vi "DriveSimulationInit.vi"() -> (1 "Module Positions":T6[](array[typedef]) {"Angle"."SIN" format="%13.4f"; "Angle"."COS" format="%13.4f"; "Angle"."VALUE" format="%13.4f"}, 2 "TravelMotorDmd":dbl, 3 "SWERVE_DRIVE_KINEMATICS":T1 {"SavedModuleStates"."Angle"."SIN" format="%13.4f"; "SavedModuleStates"."Angle"."COS" format="%13.4f"; "SavedModuleStates"."Angle"."VALUE" format="%13.4f"; "PrevCoR"."Y" format="%14.3f"; "PrevCoR"."X" format="%14.3f"; "Modules"."Y" format="%14.3f"; "Modules"."X" format="%14.3f"})   [LabVIEW 2023]
uses:
  <vilib>/Rock Robotics/WPI/ThirdParty/JAS_Junk/TrajLib/Trajectory_Library.lvlib
  DriveGlobal.vi
  <vilib>/Rock Robotics/WPI/ThirdParty/JAS_Junk/TrajLib/TypeDef/ROTATION2D.ctl
  <vilib>/Rock Robotics/WPI/ThirdParty/JAS_Junk/TrajLib/TypeDef/SWERVE_DRIVE_MODULE_POSITION.ctl
  <vilib>/Analysis/Matrix/Datatypes/RealMatrix.ctl
  <vilib>/Analysis/Matrix/NI_Matrix.lvlib
  <vilib>/Rock Robotics/WPI/ThirdParty/JAS_Junk/TrajLib/TypeDef/TRANSLATION2D.ctl
  <vilib>/Rock Robotics/WPI/ThirdParty/JAS_Junk/TrajLib/TypeDef/SWERVE_DRIVE_MODULE_STATE.ctl
  <vilib>/Rock Robotics/WPI/ThirdParty/JAS_Junk/TrajLib/TypeDef/SWERVE_DRIVE_KINEMATICS.ctl
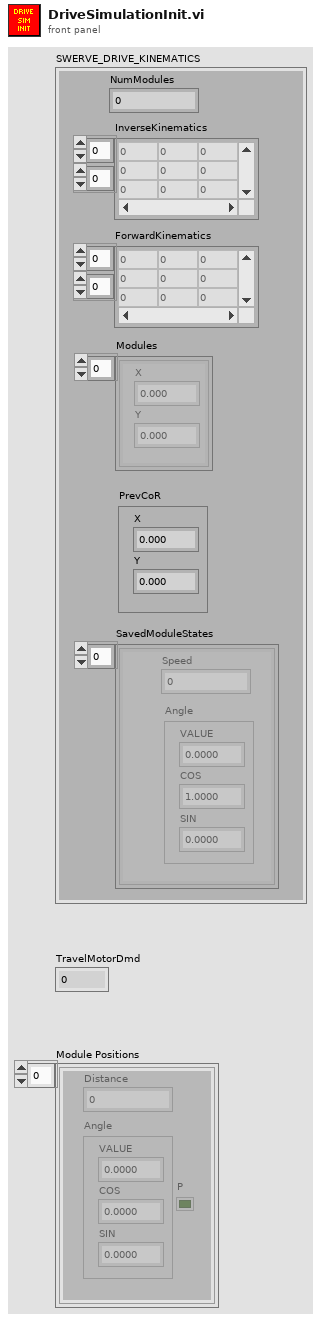
[diagram p1: front panel]
types:
  T1 = typedef "Trajectory_Library.lvlib/SWERVE_DRIVE_KINEMATICS.ctl" = cluster{"NumModules":i32, "InverseKinematics":T2, "ForwardKinematics":T2, "Modules":T3[], "PrevCoR":T3, "SavedModuleStates":T4[]}
  T2 = typedef "NI_Matrix.lvlib/RealMatrix.ctl" = dbl[][]
  T3 = typedef "Trajectory_Library.lvlib/TRANSLATION2D.ctl" = cluster{"X":dbl, "Y":dbl}
  T4 = typedef "Trajectory_Library.lvlib/SWERVE_DRIVE_MODULE_STATE.ctl" = cluster{"Speed":dbl, "Angle":T5}
  T5 = typedef "Trajectory_Library.lvlib/ROTATION2D.ctl" = cluster{"VALUE":dbl, "COS":dbl, "SIN":dbl}
  T6 = typedef "Trajectory_Library.lvlib/SWERVE_DRIVE_MODULE_POSITION.ctl" = cluster{"Distance":dbl, "Angle":T5, "P":bool}
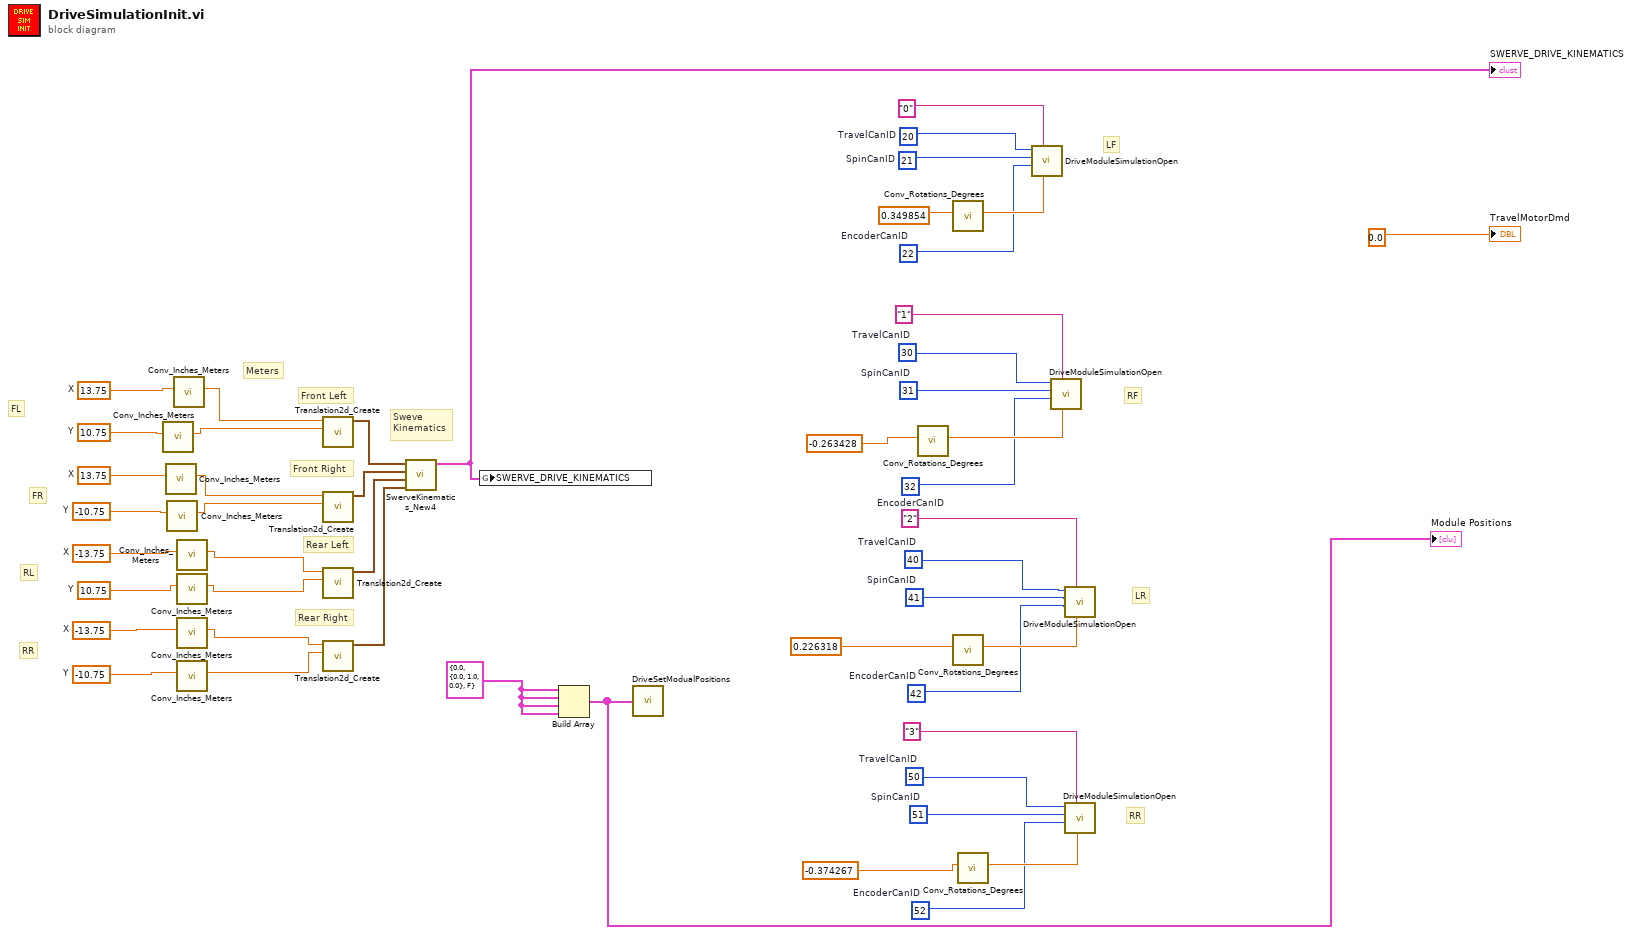
[diagram p0: block diagram]
diagram:
  w36 = u8 50  # TravelCanID
  w37 = u8 51  # SpinCanID
  w38 = u8 52  # EncoderCanID
  w33 = u8 40  # TravelCanID
  w34 = u8 41  # SpinCanID
  w35 = u8 42  # EncoderCanID
  w30 = u8 30  # TravelCanID
  w31 = u8 31  # SpinCanID
  w32 = u8 32  # EncoderCanID
  w29 = u8 20  # TravelCanID
  w28 = u8 21  # SpinCanID
  w27 = u8 22  # EncoderCanID
  w21 = T6 {"Distance"=0.0, "Angle"={"VALUE"=0.0, "COS"=1.0, "SIN"=0.0}, "P"=FALSE} ("SWERVE_DRIVE_MODULE_POSITION")
  w19 = -13.75  # X
  w20 = -10.75  # Y
  w17 = -13.75  # X
  w18 = 10.75  # Y
  w15 = 13.75  # X
  w16 = -10.75  # Y
  w13 = 13.75  # X
  w14 = 10.75  # Y
  # "RR"
  # "LR"
  # "RF"
  # "LF"
  # "RR"
  # "RL"
  # "FR"
  # "FL"
  # "Meters"
  # "Sweve\nKinematics"
  # "Rear Right"
  # "Rear Left"
  # "Front Right"
  # "Front Left"
  n1 = call <vilib>:"Conv_Inches_Meters.vi"("INCH"=w14) -> ("Meters"=w11:dbl)  [unwired: 10 in]
  n2 = call <vilib>:"Conv_Inches_Meters.vi"("INCH"=w15) -> ("Meters"=w10:dbl)  [unwired: 10 in]
  n3 = call <vilib>:"Conv_Inches_Meters.vi"("INCH"=w16) -> ("Meters"=w9:dbl)  [unwired: 10 in]
  n4 = call <vilib>:"Conv_Inches_Meters.vi"("INCH"=w13) -> ("Meters"=w12:dbl)  [unwired: 10 in]
  n5 = call <vilib>:"Conv_Inches_Meters.vi"("INCH"=w17) -> ("Meters"=w8:dbl)  [unwired: 10 in]
  n6 = call <vilib>:"Conv_Inches_Meters.vi"("INCH"=w18) -> ("Meters"=w7:dbl)  [unwired: 10 in]
  n7 = call <vilib>:"Conv_Inches_Meters.vi"("INCH"=w19) -> ("Meters"=w5:dbl)  [unwired: 10 in]
  n8 = call <vilib>:"Conv_Inches_Meters.vi"("INCH"=w20) -> ("Meters"=w6:dbl)  [unwired: 10 in]
  n9 = call <vilib>:"Translation2d_Create.vi"("Y"=w11, "X"=w12) -> ("TRANSLATION"=w4:T3)  [unwired: 9 in]
  n10 = call <vilib>:"Translation2d_Create.vi"("Y"=w9, "X"=w10) -> ("TRANSLATION"=w3:T3)  [unwired: 9 in]
  n11 = call <vilib>:"Translation2d_Create.vi"("Y"=w7, "X"=w8) -> ("TRANSLATION"=w2:T3)  [unwired: 9 in]
  n12 = call <vilib>:"Translation2d_Create.vi"("Y"=w6, "X"=w5) -> ("TRANSLATION"=w1:T3)  [unwired: 9 in]
  n13 = call <vilib>:"SwerveKinematics_New4.vi"("wheel 3"=w1, "wheel 2"=w2, "wheel 1"=w3, "wheel 0"=w4) -> ("SWERVE_DRIVE_KINEMATICS"=w47:T1)  [unwired: 7 in]
  "SWERVE_DRIVE_KINEMATICS" <- w47
  n14 = global write "DriveGlobal.vi" "SWERVE_DRIVE_KINEMATICS"(w47) -> ()
  n15 = Build Array(w21, w21, w21, w21) -> (w48:T6[])
  "Module Positions" <- w48
  n16 = call "DriveSetModualPositions.vi"("Swerve_Drive_Modual_Position"=w48) -> ()  [unwired: 11 in]
  n17 = call <vilib>:"Conv_Rotations_Degrees.vi"("Rotations"=-0.263428 ("Magnet Offset (Degrees)")) -> ("Degrees"=w42:dbl)  [unwired: 10 in]
  n18 = call <vilib>:"Conv_Rotations_Degrees.vi"("Rotations"=0.349854 ("Magnet Offset (Degrees)")) -> ("Degrees"=w39:dbl)  [unwired: 10 in]
  n19 = call <vilib>:"Conv_Rotations_Degrees.vi"("Rotations"=0.226318 ("Magnet Offset (Degrees)")) -> ("Degrees"=w44:dbl)  [unwired: 10 in]
  n20 = call <vilib>:"Conv_Rotations_Degrees.vi"("Rotations"=-0.374267 ("Magnet Offset (Degrees)")) -> ("Degrees"=w46:dbl)  [unwired: 10 in]
  n21 = call "DriveModuleSimulationOpen.vi"("Magnet Offset (Degrees)"=w39, "ModualNamePrefix"="0", "EncoderCanID"=w27, "SpinCanID"=w28, "TravelCanID"=w29) -> ()  [unwired: 6 in, 1 out]
  n22 = call "DriveModuleSimulationOpen.vi"("Magnet Offset (Degrees)"=w42, "ModualNamePrefix"="1", "EncoderCanID"=w32, "SpinCanID"=w31, "TravelCanID"=w30) -> ()  [unwired: 6 in, 1 out]
  n23 = call "DriveModuleSimulationOpen.vi"("Magnet Offset (Degrees)"=w44, "ModualNamePrefix"="2", "EncoderCanID"=w35, "SpinCanID"=w34, "TravelCanID"=w33) -> ()  [unwired: 6 in, 1 out]
  n24 = call "DriveModuleSimulationOpen.vi"("Magnet Offset (Degrees)"=w46, "ModualNamePrefix"="3", "EncoderCanID"=w38, "SpinCanID"=w37, "TravelCanID"=w36) -> ()  [unwired: 6 in, 1 out]
  "TravelMotorDmd" <- 0.0 ("TravelMotorDmd")
